vi "calc_NH_vector.vi"(6 "current pipette location (px)":dbl[](array[numeric]), 7 "which manipulator":T3(ring), 8 "cell tracker movement options":T1={"step down by (steps)"=10.0, "descend threshold (px)"=10.0, "step XY by (steps)"=10.0} {"descend threshold (px)" format="%#_13g"; "step down by (steps)" format="%#_13g"}, 9 "transform cluster + actuator":T2, 11 "cell centroid (px)":dbl[](array[numeric])) -> (3 "rel move vector (steps)":dbl[](array[numeric]))   [LabVIEW 2015]
uses:
  <vilib>/Analysis/NI_AALBase.lvlib
  <vilib>/Analysis/baseanly.llb/Unit Vector (DBL).vi
  <vilib>/Analysis/_algsub.llb/Vector Norm Type.ctl
  <vilib>/Analysis/NI_AALPro.lvlib
  pipette cleaning/pressure box/cleaning_soft/controls/actuator_type.ctl
  pipette cleaning/pressure box/cleaning_soft/controls/actuator_cluster.ctl
  machine_vision/coordinate model vis/transform_properties_actuators.ctl
  machine_vision/controls/transform_cluster_actuator.ctl
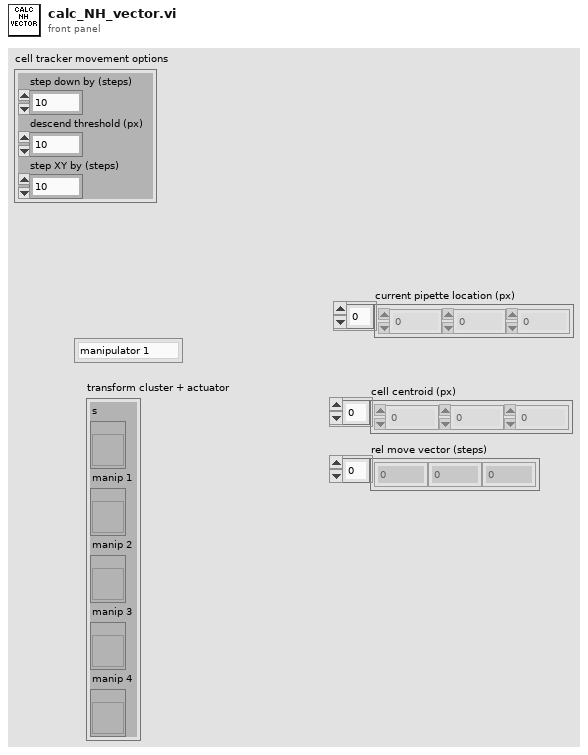
[diagram p1: front panel]
types:
  T1 = cluster{"step down by (steps)":dbl, "descend threshold (px)":dbl, "step XY by (steps)":dbl}
  T2 = typedef "transform_cluster_actuator.ctl" = cluster{"s":refnum<vi>, "manip 1":refnum<vi>, "manip 2":refnum<vi>, "manip 3":refnum<vi>, "manip 4":refnum<vi>}
  T3 = enum16{"manipulator 1", "manipulator 2", "manipulator 3", "manipulator 4"}
  T4 = typedef "NI_AALPro.lvlib/Vector Norm Type.ctl" = u16
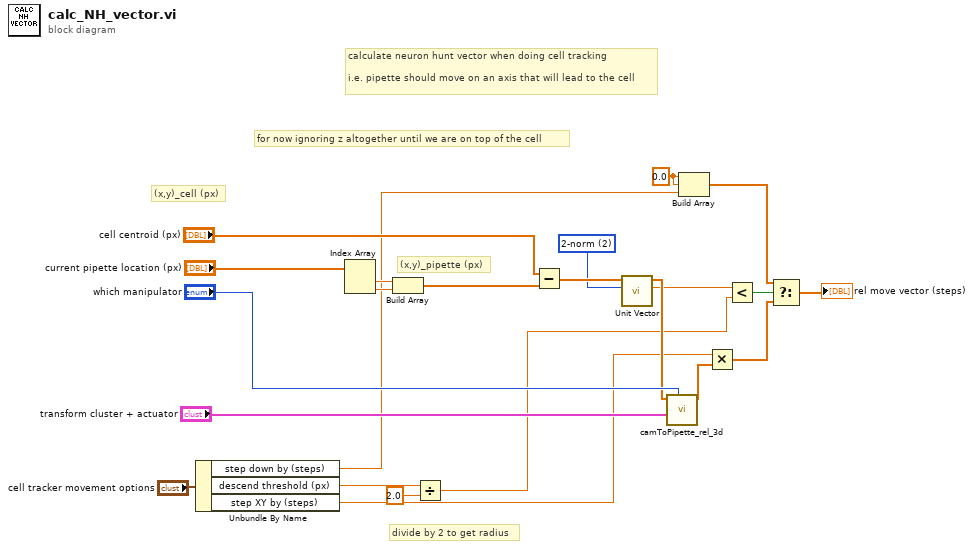
[diagram p0: block diagram]
diagram:
  w14 = 0.0 ("element")
  w21 = T4 2 items=["1-norm"=1, "2-norm"=2, "Inf-norm"=3, "-Inf-norm"=4, "User Defined"=5] ("norm type")
  # "divide by 2 to get radius"
  # "(x,y)_pipette (px)"
  # "(x,y)_cell (px)"
  # "for now ignoring z altogether until we are on top of the cell"
  # "calculate neuron hunt vector when doing cell tracking\n\ni.e. pipette should move on an axis that will lead to the cell"
  n1 = Unbundle By Name("cell tracker movement options") -> ("step down by (steps)"=w5:dbl, "descend threshold (px)"=w3:dbl, "step XY by (steps)"=w4:dbl)
  n2 = Index Array(array="current pipette location (px)") -> (element #1=w9:dbl, element #2=w8:dbl)  [unwired: 2 in]
  n3 = Build Array(w9, w8) -> (w7:dbl[])
  n4 = Divide(x=w3, y=2.0) -> (x/y=w2:dbl)
  n5 = Subtract(x="cell centroid (px)", y=w7) -> (x-y=w22:dbl[])
  n6 = call-poly <vilib>:"Unit Vector.vi"("norm type"=w21, "Input Vector"=w22) -> ("norm"=w16:dbl, "Unit Vector"=w17:dbl[])  [unwired: 7 in, 1 out]
  n7 = call "camToPipette_rel_3d.vi"("which manipulator"="which manipulator", "transform cluster + actuator"="transform cluster + actuator", "rel cam (px)"=w17) -> ("rel pipette (steps)"=w18:dbl[])  [unwired: 8 in]
  n8 = Build Array(w14, w14, w5) -> (w13:dbl[])
  n9 = Multiply(x=w4, y=w18) -> (x*y=w12:dbl[])
  n10 = Less?(x=w16, y=w2) -> (x < y?=w15:bool)
  n11 = Select(t=w13, s=w15, f=w12) -> (s? t:f=→"rel move vector (steps)":dbl[])
